vi "Exfo Unit Test.vi"() -> ()   [LabVIEW 2018]
uses:
  bc37d0f5-e284-46b3-94d6-c408141ba29d.vi
  8482574f-6e04-49c0-8121-85397b976351.vi
  PPLs/EXFO/Parent/EXFO.lvlibp/EXFO.lvclass
panel:
  out "Attenuation Read":dbl
  out "Shutter Status":bool
  in  "Shutter":bool
  in  "Attenuation":dbl(slide) scale=1.052..73.567
  out "Power (dBm)":dbl
  out "Power (W)":dbl
  out "EXFO Connected":bool
  in  "PPLs Folder Path":path
  in  "INI File Path":path
  in  "stop":bool
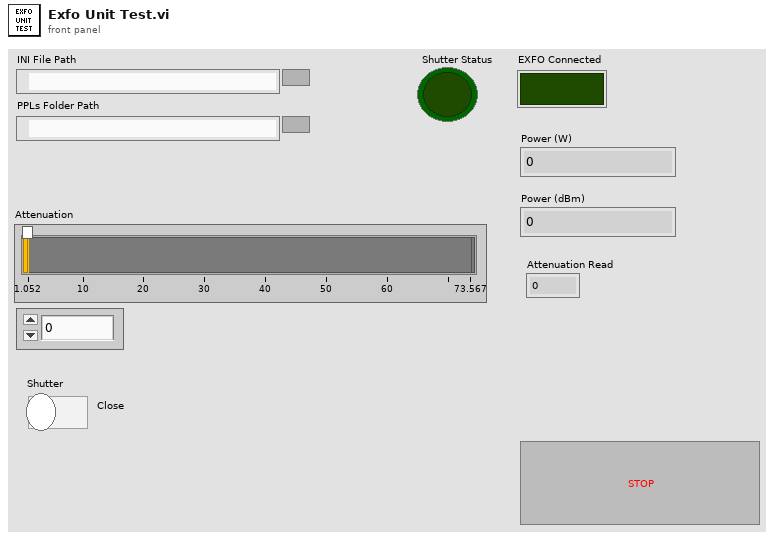
[diagram p1: front panel]
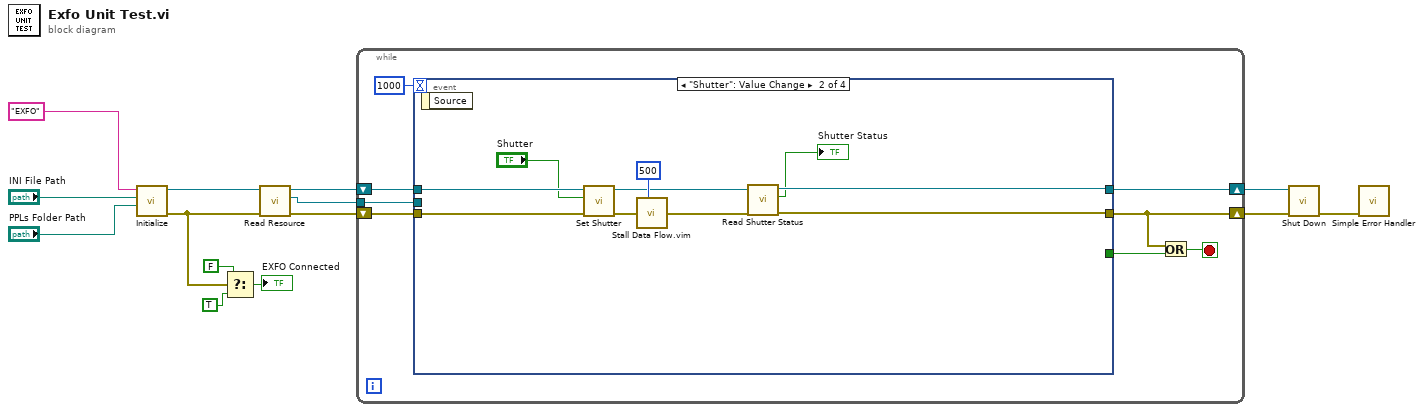
[diagram p0: block diagram]
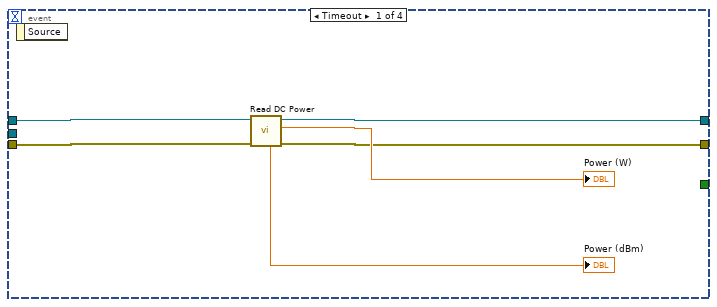
[diagram p2: hidden frame]
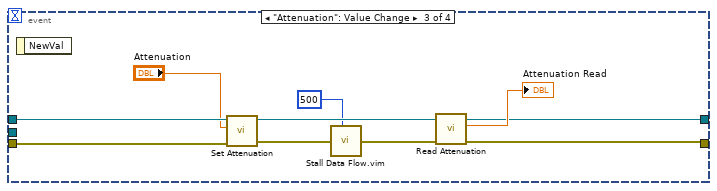
[diagram p3: hidden frame]
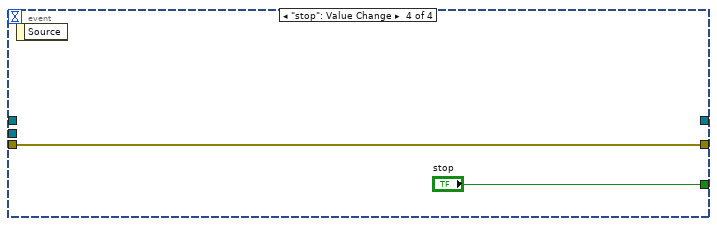
[diagram p4: hidden frame]
diagram:
  n1 = call "Initialize.vi"("PPLs Folder Path"="PPLs Folder Path", "INI File Path"="INI File Path", "Device"="EXFO") -> ("error out"=w3:errorcluster, "EXFO out"=w5:refnum<class "EXFO.lvclass">)  [unwired: 7 in]
  n2 = Select(t=FALSE, s=w3, f=TRUE) -> (s? t:f=→"EXFO Connected":bool)
  n3 = call "Read Resource.vi"("error in (no error)"=w3, "EXFO in"=w5) -> ("error out"=w4:errorcluster, "Resource"=w1:refnum<visa-resource-name>, "EXFO out"=w2:refnum<class "EXFO.lvclass">)  [unwired: 7 in]
  n4 = while {
    shift-right: [w17] -> w9
    shift-left: w2 -> [w16]
    shift-right: [w20] -> w14
    shift-left: w4 -> [w21]
    tunnel: w1 -> [w15]
    stop <- w19 stop-if-true
    n5 = event shown="[1] \"Shutter\": Value Change" {
      selector: _ -> [_ _ _ _]
      dyn-events: _ -> [_ _ _ _]
      timeout: 1000 -> [_ _ _ _]
      tunnel: w21 -> [w28 w37 w47 w50]
      tunnel: [w23 w30 w42 w50] -> w20
      tunnel: [_ _ _ "stop"] -> w18
      tunnel: [w24 w31 w41 _] -> w17
      tunnel: w16 -> [w25 w38 w48 _]
      tunnel: w15 -> [_ _ _ _]
      event Timeout {
        n6 = event-data() -> ()  [unwired: 1 in, 1 out]
        n7 = call-dynamic "Read DC Power.vi"("error in (no error)"=w28, "EXFO in"=w25) -> ("error out"=w23:errorcluster, "Power (uW)"=→"Power (W)":dbl, "EXFO out"=w24:refnum<class "EXFO.lvclass">, "Power dBm"=→"Power (dBm)":dbl)  [unwired: 6 in]
      }
      event "Shutter": Value Change {
        n8 = event-data() -> ()  [unwired: 1 in, 1 out]
        n9 = call-dynamic "Set Shutter.vi"("error in (no error)"=w37, "Shutter"="Shutter", "EXFO in"=w38) -> ("error out"=w35:errorcluster, "EXFO out"=w33:refnum<class "EXFO.lvclass">)  [unwired: 7 in]
        n10 = call "Stall Data Flow.vim"("value in"=w35, "milliseconds to wait"=u32 500) -> ("value out"=w32:errorcluster)  [unwired: 1 out]
        n11 = call-dynamic "Read Shutter Status.vi"("error in (no error)"=w32, "EXFO in"=w33) -> ("error out"=w30:errorcluster, "Shutter Status"=→"Shutter Status":bool, "EXFO out"=w31:refnum<class "EXFO.lvclass">)  [unwired: 7 in]
      }
      event "Attenuation": Value Change {
        n12 = event-data() -> ()  [unwired: 1 in, 1 out]
        n13 = call-dynamic "Set Attenuation.vi"("error in (no error)"=w47, "Attenuation"="Attenuation", "EXFO in"=w48) -> ("error out"=w43:errorcluster, "EXFO out"=w44:refnum<class "EXFO.lvclass">)  [unwired: 7 in]
        n14 = call "Stall Data Flow.vim"("value in"=w43, "milliseconds to wait"=u32 500) -> ("value out"=w40:errorcluster)  [unwired: 1 out]
        n15 = call-dynamic "Read Attenuation.vi"("error in (no error)"=w40, "EXFO in"=w44) -> ("error out"=w42:errorcluster, "Attenuation"=→"Attenuation Read":dbl, "EXFO out"=w41:refnum<class "EXFO.lvclass">)  [unwired: 7 in]
      }
      event "stop": Value Change {
        n16 = event-data() -> ()  [unwired: 1 in, 1 out]
      }
    }
    n17 = Or(x=w20, y=w18) -> (x .or. y?=w19:bool)
  }
  n18 = call "Shut Down.vi"("error in"=w14, "EXFO in"=w9) -> ("error out"=w13:errorcluster)  [unwired: 9 in]
  n19 = call <vilib>:"Simple Error Handler.vi"("error in (no error)"=w13) -> ()  [unwired: 4 in, 5 out]
